vi "SetProjectNumber.vi"() -> ()   [LabVIEW 2010]
panel:
  in  "ProjectNumberToSet":string
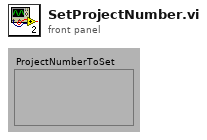
[diagram p1: front panel]
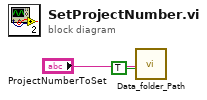
[diagram p0: block diagram]
diagram:
  n1 = call "Data_folder_Path.vi"("ProjectNumberIn"="ProjectNumberToSet", "SetProjectNumber"=TRUE) -> ()  [unwired: 3 in, 1 out]
